vi "SW_Add_or_Modify_Reward_Condition.vi"(6 "IO parameters cluster":T1, 7 "Add or Modify?":enum16{"Add", "Modify"}(ring), 8 "error in (no error)":T15, 9 "Main Tree Control in":refnum<vi>, 10 "Calibration parameters":T13={"Timing calibration sw/hw"=1.0, "True FPS"=80.0, "True frame time, s"=0.0125, "Disp. calibration info"=[]} {"True frame time, s" format="%.10g"; "Disp. calibration info"."Speed, µl per ms" format="%.3g"; "True FPS" format="%.10g"; "Timing calibration sw/hw" format="%.10g"}, 11 "Array of conditions in":T12 {"Specifier(s)"."Validity criteria(s)"."Validity value" min=0.0 step=0.1 format="%.2g"; "Specifier(s)"."Value" step=1.0 format="%#.2g"}) -> (0 "error out":T15, 1 "Main Tree Control out":refnum<vi>, 3 "Array of conditions out":T12 {"Specifier(s)"."Validity criteria(s)"."Validity value" min=0.0 step=0.1 format="%.2g"; "Specifier(s)"."Value" step=1.0 format="%#.2g"})   [LabVIEW 2018, in "Tracker.lvlib"]
uses:
  Tracker.lvlib
  Controls/CTL_Conditions_Array.ctl
  Controls/CTL_Conditions_Cluster.ctl
  Controls/CTL_Condition_type.ctl
  Controls/CTL_Comparison_type.ctl
  Controls/CTL_Validity_check_criteria.ctl
  Controls/CTL_Response_info.ctl
  Controls/CTL_Condition_response_type.ctl
  Controls/CTL_Reponse_port_info.ctl
  Controls/CTL_Calibration_parameters.ctl
  Controls/CTL_Dispenser_calibration_info.ctl
  Controls/CTL_IO_params_cluster.ctl
  <vilib>/Utility/miscctls.llb/LVPointTypeDef.ctl
  Controls/CTL_Conditions_build_parameters_in.ctl
panel:
  out "Local tree ref":refnum<vi>
  in  "Discard and exit":bool
  in  "Reset Button":bool
  out "Index of selected condition":i32
  out "Has been set":bool
  in  "Specifiers On/Off":T2
  in  "Save and exit":bool
  out "Validity criteria(s)":T4(array[cluster])
  out "Subcondition":T5={"Enabled"=FALSE, "Name"="", "Specifier(s)"=[], "Response"={"Response type"=enum."Air puff", "TTL port"=enum."Port 1", "TTL pulse length, ms"=0.0}, "Has been set"=FALSE} caption="Condition" {"Specifier(s)"."Validity criteria(s)"."Validity value" min=0.0 step=0.1 format="%.2g"; "Specifier(s)"."Value" step=1.0 format="%#.2g"}
  in  "TTL pulse length":dbl caption="Puff length, ms"
  in  "TTL port":T10
  in  "Response type":T9=enum."Air puff"
  in  "Valid for, units":dbl caption="Has been True for, units" format="%.2g"
  in  "Validity Enabled":bool caption="Enabled"
  in  "SC. Validity Criteria":T3 caption="Validity Criteria"
  in  "Compare against":dbl
  in  "Comparison type":T7
  in  "SubCondition type":T6
  in  "Subcondition #":i32(slide)=5 min=1 max=5 step=1 scale=5.0..1.0
  in  "Specifier(s)":T11(array[cluster])
  in  "C. Name":string caption="Condition Name"
  out "Cond. work index":i32
  in  "C. Enabled":bool caption="Enabled"
  out "Review changes before save":string(tree) caption="Reward and stimulation out"
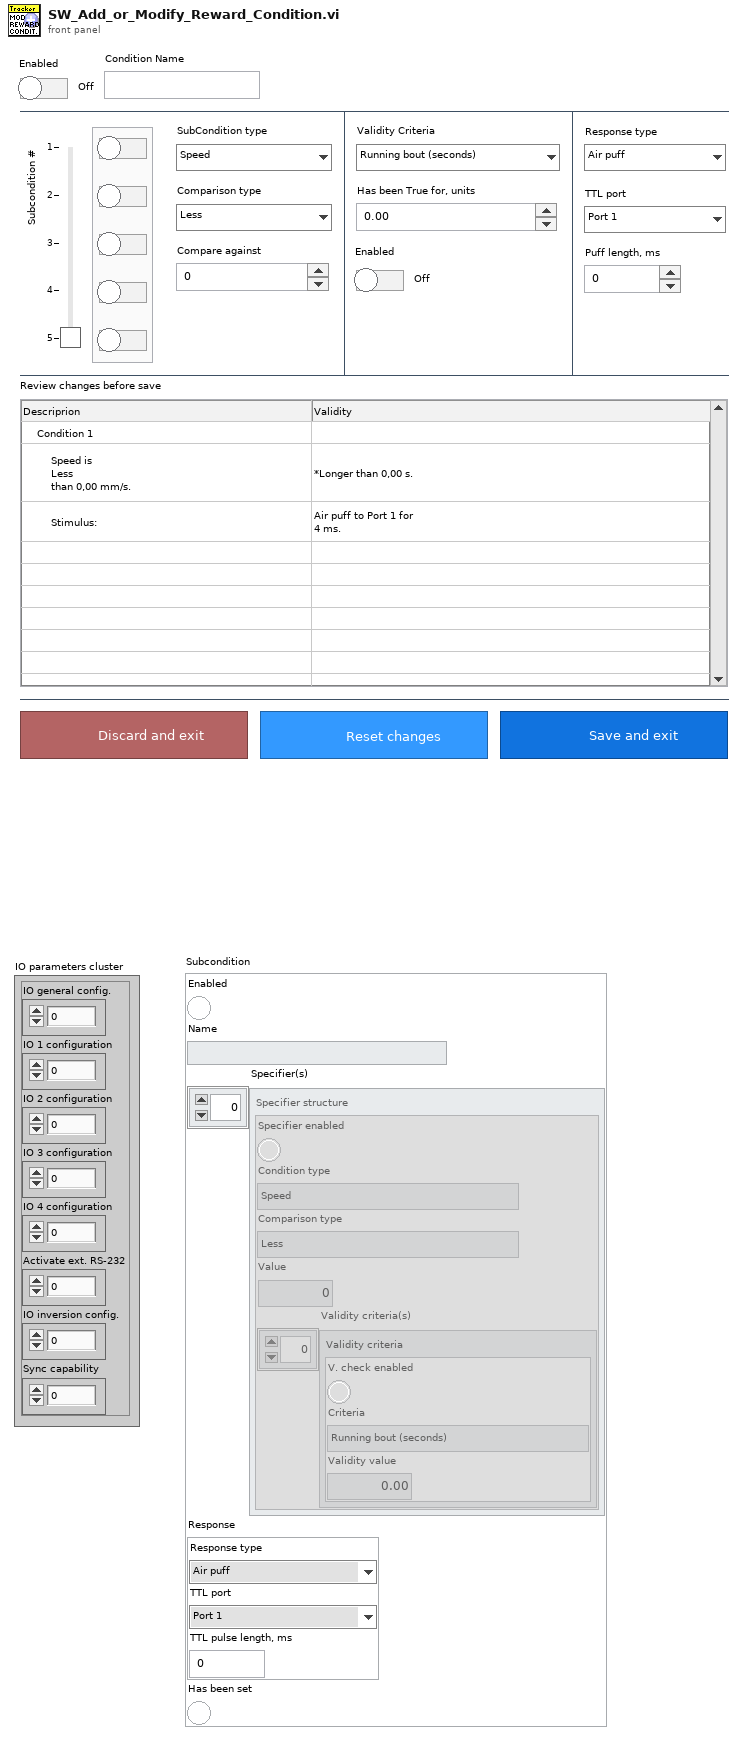
[diagram p1: front panel]
types:
  T1 = typedef "Tracker.lvlib/CTL_IO_params_cluster.ctl" = cluster{"IO general config.":u16, "IO 1 configuration":u16, "IO 2 configuration":u16, "IO 3 configuration":u16, "IO 4 configuration":u16, "Activate ext. RS-232":u16, "IO inversion config.":u16, "Sync capability":u8}
  T2 = cluster{"Specifier on/off":bool, "Specifier on/off 2":bool, "Specifier on/off 3":bool, "Specifier on/off 4":bool, "Specifier on/off 5":bool}
  T3 = typedef "Tracker.lvlib/CTL_Validity_check_criteria.ctl" = enum16{"Running bout (seconds)", "Running bout (meters)"}
  T4 = cluster{"V. check enabled":bool, "Criteria":T3, "Validity value":dbl}[]
  T5 = typedef "Tracker.lvlib/CTL_Conditions_Cluster.ctl" = cluster{"Enabled":bool, "Name":string, "Specifier(s)":cluster{"Specifier enabled":bool, "Condition type":T6, "Comparison type":T7, "Value":dbl, "Validity criteria(s)":cluster{"V. check enabled":bool, "Criteria":T3, "Validity value":dbl}[]}[], "Response":T8, "Has been set":bool}
  T6 = typedef "Tracker.lvlib/CTL_Condition_type.ctl" = enum16{"Speed", "Zone", "Angle to wall"}
  T7 = typedef "Tracker.lvlib/CTL_Comparison_type.ctl" = enum16{"Less", "Less or Equal", "Equal", "Greater or Equal", "Greater", "Not Equal"}
  T8 = typedef "CTL_Response_info.ctl" = cluster{"Response type":T9, "TTL port":T10, "TTL pulse length, ms":dbl}
  T9 = typedef "Tracker.lvlib/CTL_Condition_response_type.ctl" = enum16{"None", "Air puff", "Liquid reward"}
  T10 = typedef "CTL_Reponse_port_info.ctl" = enum16{"Port 1", "Port 2", "Port 3", "Port 4"}
  T11 = cluster{"Specifier enabled":bool, "Condition type":T6, "Comparison type":T7, "Value":dbl, "Validity criteria(s)":cluster{"V. check enabled":bool, "Criteria":T3, "Validity value":dbl}[]}[]
  T12 = typedef "Tracker.lvlib/CTL_Conditions_Array.ctl" = T5[]
  T13 = typedef "Tracker.lvlib/CTL_Calibration_parameters.ctl" = cluster{"Timing calibration sw/hw":dbl, "True FPS":dbl, "True frame time, s":dbl, "Disp. calibration info":T14}
  T14 = typedef "Tracker.lvlib/CTL_Dispenser_calibration_info.ctl" = cluster{"Channel":u8, "Speed, µl per ms":dbl}[]
  T15 = cluster{"Boolean Round":bool, "code":i32, "source":string}
  T16 = typedef "LVPointTypeDef.ctl" = cluster{"Horizontal":i16, "Vertical":i16}
  T17 = typedef "Tracker.lvlib/CTL_Conditions_build_parameters_in.ctl" = cluster{"TreeControl in":refnum<vi>, "TTL pulse length ref in":refnum<vi>, "Array of conditions in":T12, "Condition working index":i32, "Subcondition #":i32, "Calibration parameters":T13}
  T18 = typedef "Tracker.lvlib/CTL_Conditions_build_parameters_out.ctl" = cluster{"TreeControl ref out":refnum<vi>, "SubCondition":T5, "C. Enabled":bool, "C. Name":string, "Specifier(s)":cluster{"Specifier enabled":bool, "Condition type":T6, "Comparison type":T7, "Value":dbl, "Validity criteria(s)":cluster{"V. check enabled":bool, "Criteria":T3, "Validity value":dbl}[]}[], "Has been set":bool, "Condition type":T6, "Comparison type":T7, "Compare against value":dbl, "Validity criteria(s)":cluster{"V. check enabled":bool, "Criteria":T3, "Validity value":dbl}[], "V. check enabled":bool, "Validity criteria":T3, "Validity value":dbl, "Specifiers On/Off":cluster{"[0]":bool, "[1]":bool, "[2]":bool, "[3]":bool, "[4]":bool}, "Response type":T9, "TTL port":T10, "TTL pulse length, ms out":dbl}
  T19 = cluster{"[0]":bool, "[1]":bool, "[2]":bool, "[3]":bool, "[4]":bool}
  T20 = cluster{"Specifier enabled":bool, "Condition type":T6, "Comparison type":T7, "Value":dbl, "Validity criteria(s)":cluster{"V. check enabled":bool, "Criteria":T3, "Validity value":dbl}[]}
  T21 = cluster{"V. check enabled":bool, "Criteria":T3, "Validity value":dbl}
  T22 = cluster{"Specifiers On/Off[0]":bool, "Specifiers On/Off[1]":bool, "Specifiers On/Off[2]":bool, "Specifiers On/Off[3]":bool, "Specifiers On/Off[4]":bool}
  T23 = cluster{"Validity Enabled":bool, "SC. Validity Criteria":T3, "Valid for, units":dbl}
  T24 = cluster{"Response type":T9, "TTL port":T10, "TTL pulse length, ms out":dbl}
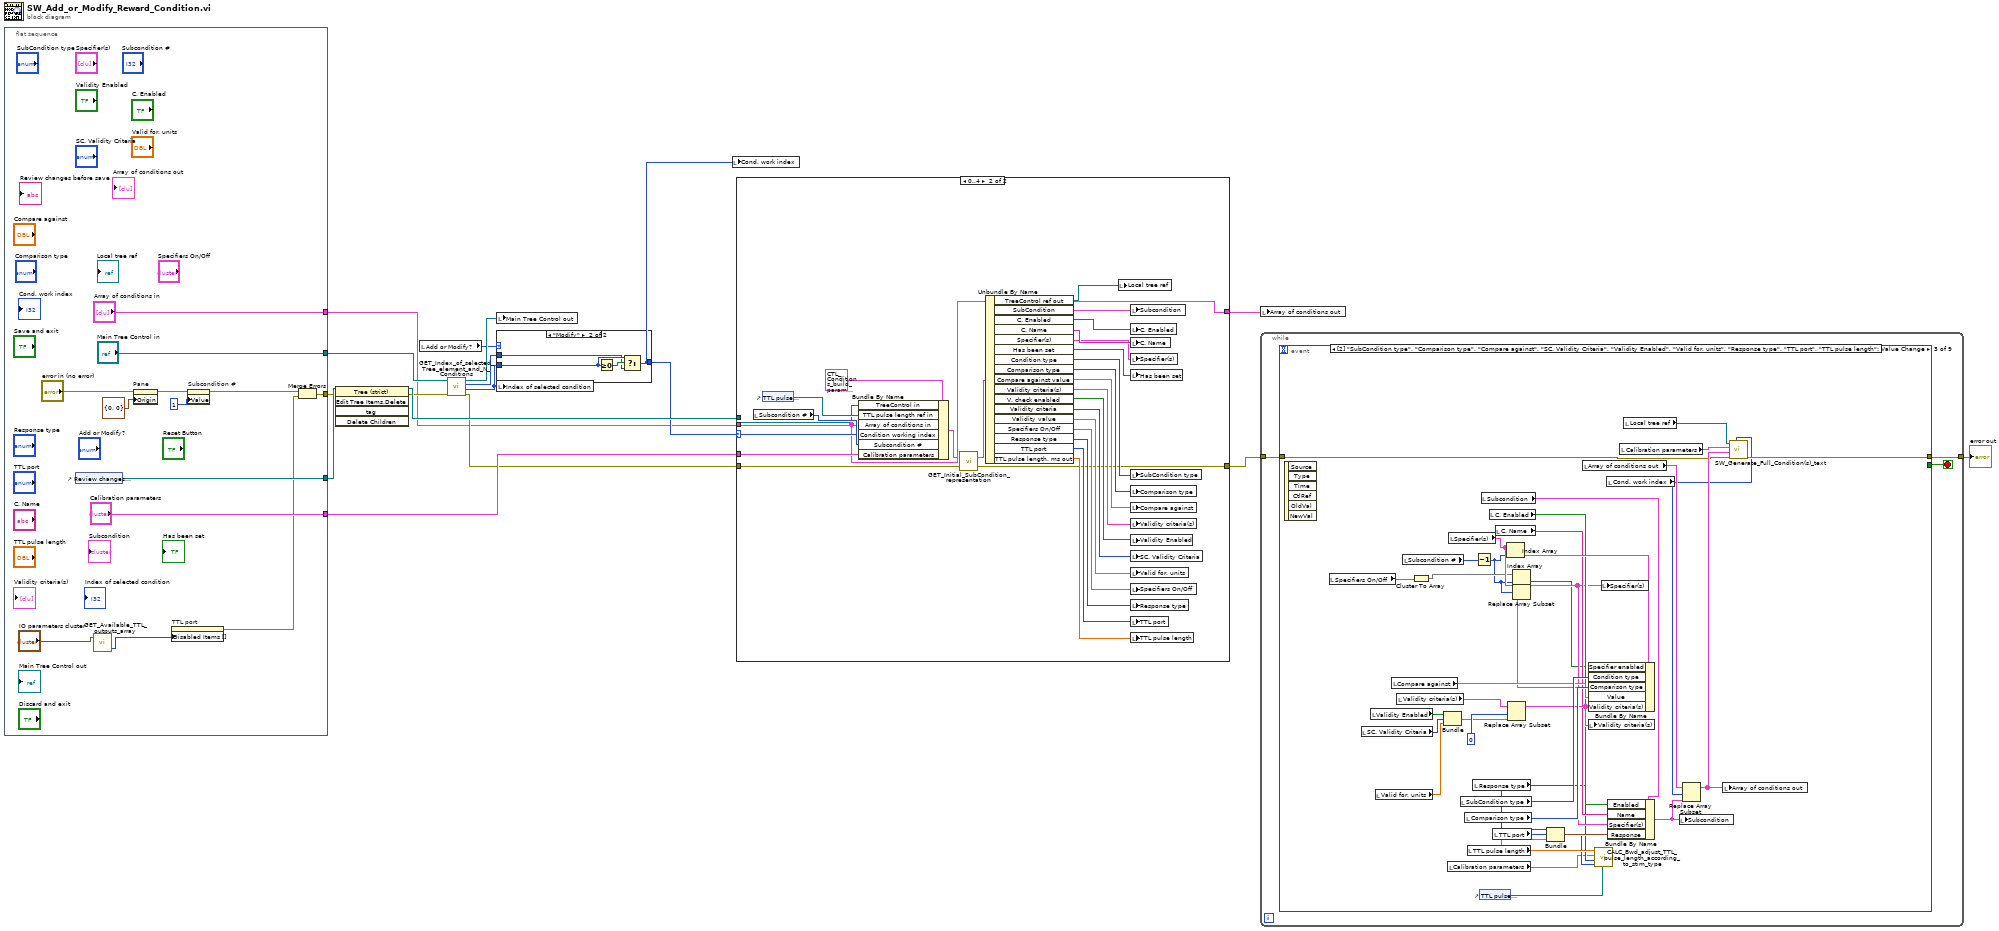
[diagram p0: block diagram]
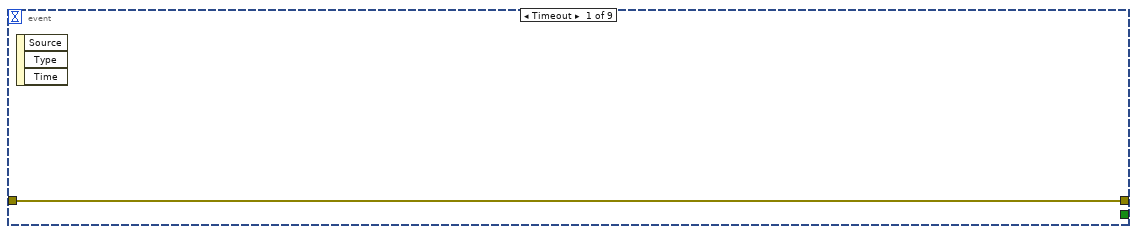
[diagram p4: hidden frame]
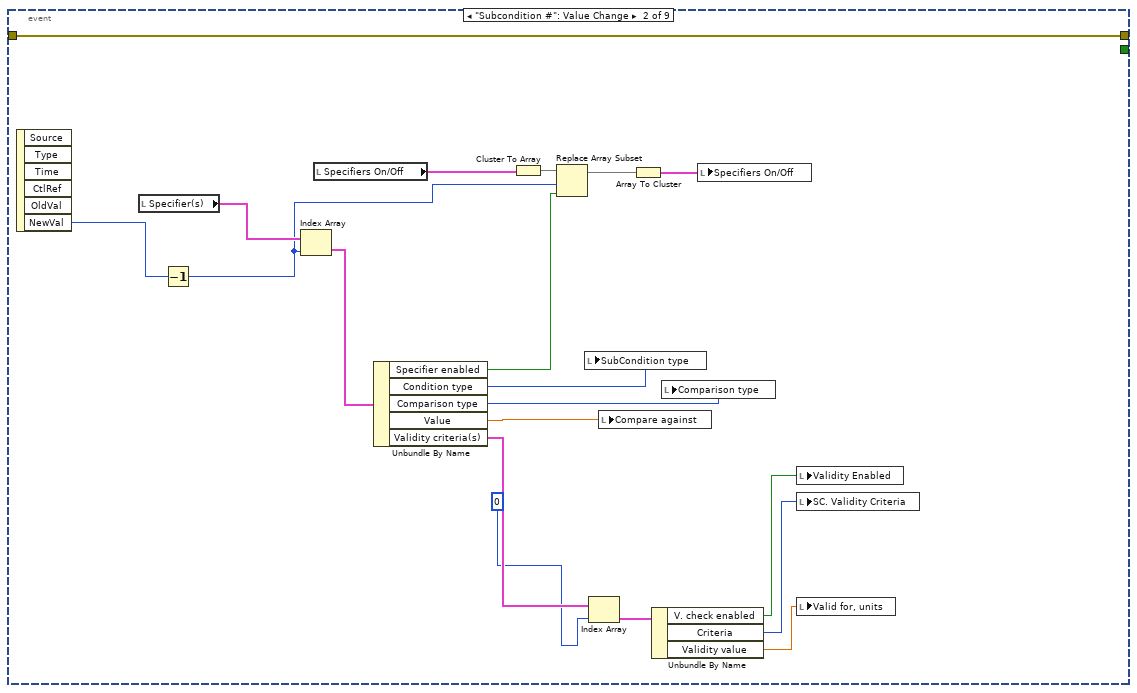
[diagram p5: hidden frame]
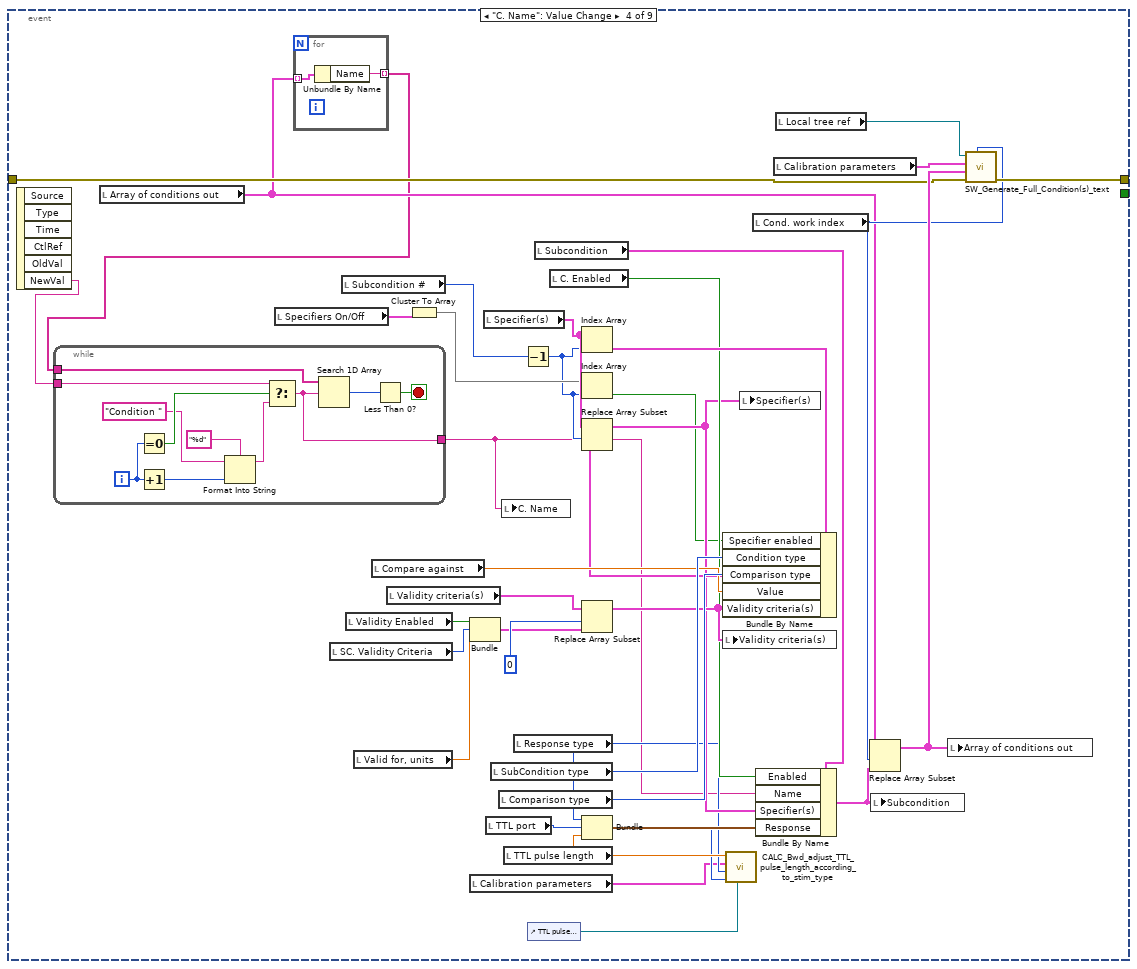
[diagram p6: hidden frame]
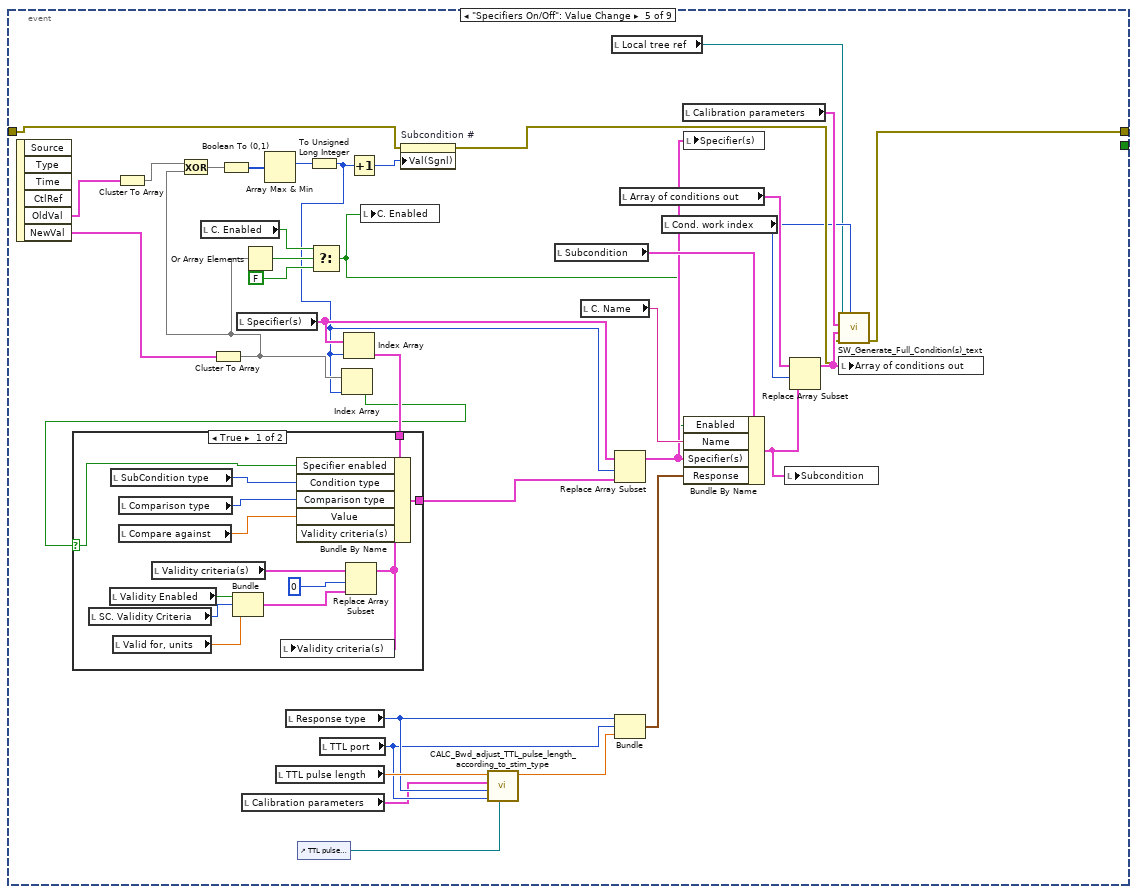
[diagram p7: hidden frame]
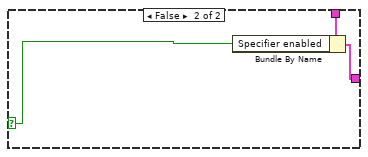
[diagram p8: hidden frame]
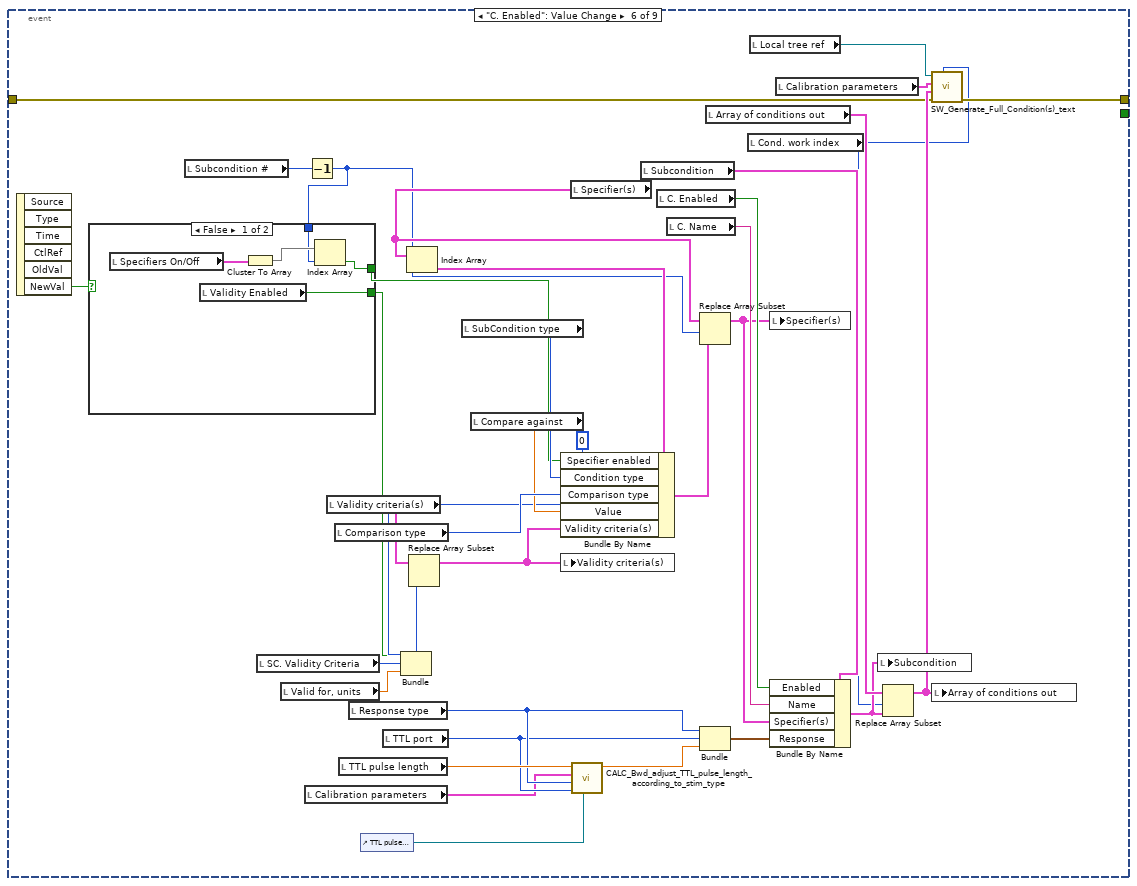
[diagram p9: hidden frame]
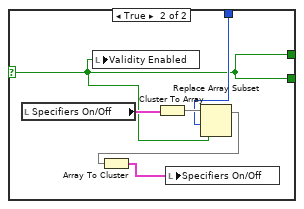
[diagram p10: hidden frame]
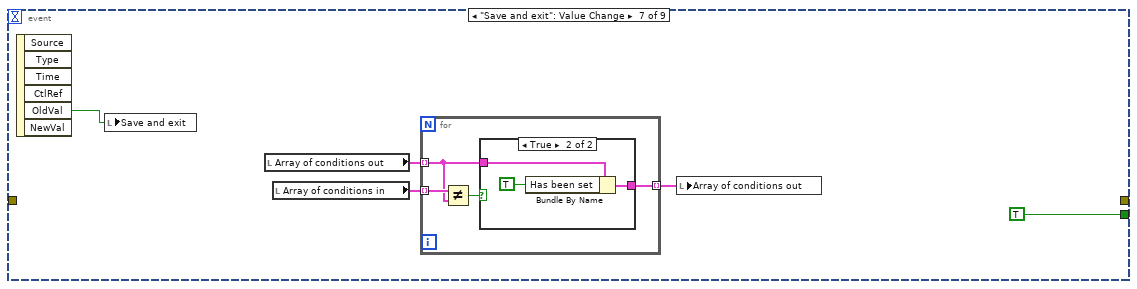
[diagram p11: hidden frame]
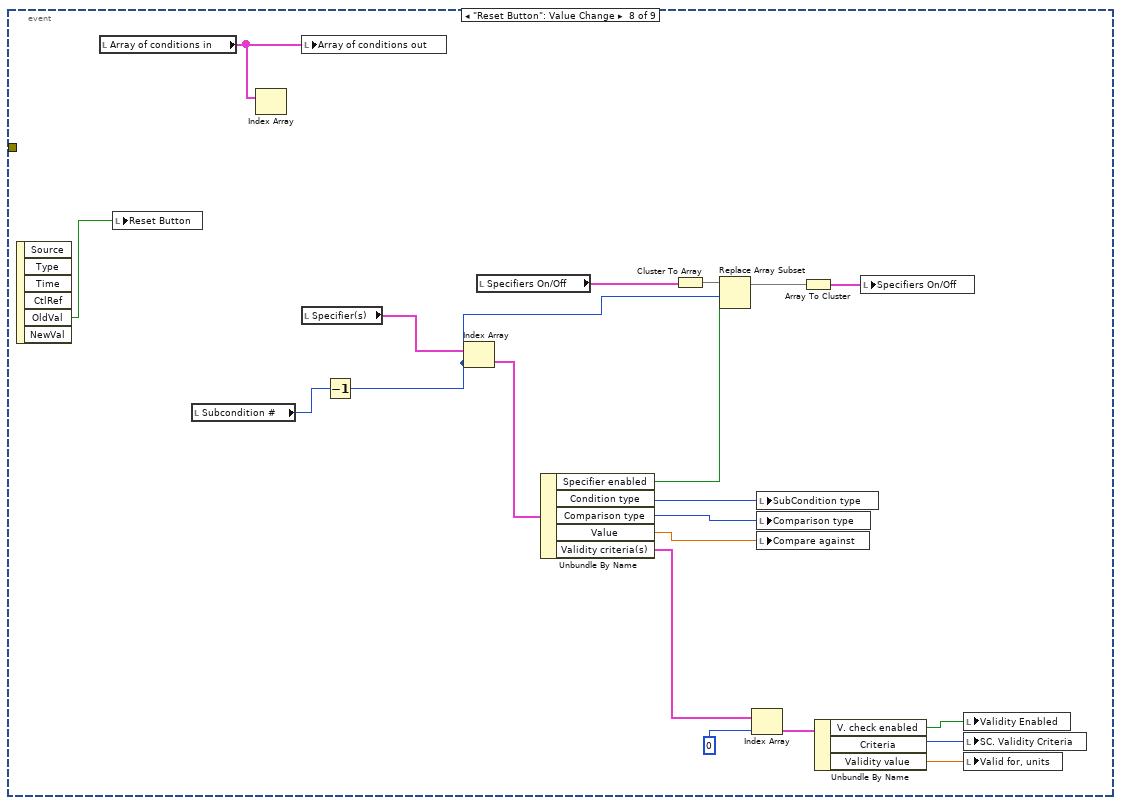
[diagram p13: hidden frame]
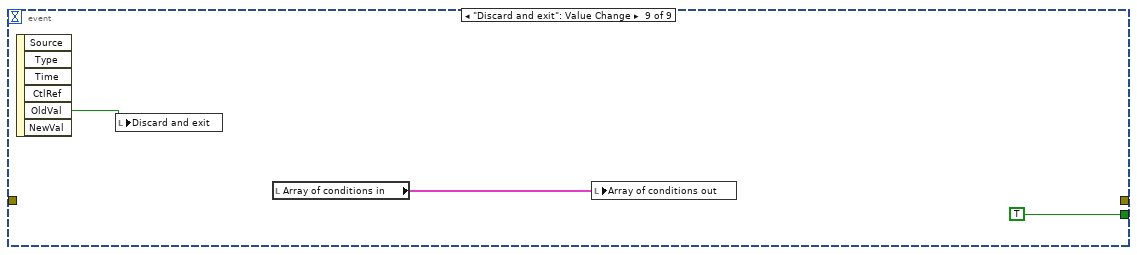
[diagram p14: hidden frame]
diagram:
  n1 = flat-sequence {
    tunnel: [w19] -> w14
    tunnel: [w27] -> w15
    tunnel: ["Main Tree Control in"] -> w4
    tunnel: ["Array of conditions in"] -> w1
    tunnel: ["Calibration parameters"] -> w12
    frame #0 {
      n2 = control-ref of="Review changes before save"() -> (w27:refnum<vi>)
      n3 = call "GET_Available_TTL_outputs_array.vi"("IO parameters cluster"="IO parameters cluster") -> ("Disabled items"=w17:i32[])  [unwired: 2 in, 1 out]
      n4 = property on="Pane" class="Pane"(error in="error in (no error)", "Origin"=T16 {"Horizontal"=0, "Vertical"=0}) -> (error out=w23:errorcluster)  [unwired: 1 in, 1 out]
      n5 = property on="TTL port" class="Enum (strict)"("Disabled Items []"=w17) -> (error out=w18:errorcluster)  [unwired: 2 in, 1 out]
      n6 = property on="Subcondition #" class="Slide (strict)"(error in=w23, "Value"=1 ("Subcondition #")) -> (error out=w22:errorcluster)  [unwired: 1 in, 1 out]
      n7 = Merge Errors(w22, w18) -> (w19:errorcluster)
    }
  }
  n8 = invoke class="Tree (strict)" method="Edit Tree Items.Delete"(reference=w15, error in=w14) -> (reference out=w11:refnum<vi>, error out=w5:errorcluster)  [unwired: 3 in, 3 out]
  n9 = local read "Add or Modify?"() -> (w7:enum16{"Add", "Modify"})
  n10 = call "GET_Index_of_selected_Tree_element_and_N_Conditions.vi"("error in (no error)"=w5, "TreeControl in"=w4) -> ("error out"=w8:errorcluster, "Index of selected element"=w2:i32, "Amount of conditions"=w3:i32, "TreeControl out"=w9:refnum<vi>)  [unwired: 6 in]
  n11 = local write "Main Tree Control out"(w9) -> ()
  n12 = case shown="\"Modify\"" w7 {
    tunnel: w3 -> [w30 w31]
    tunnel: w2 -> [_ w32]
    tunnel: [w30 w34] -> w6
    frame "Add", Default {
    }
    frame "Modify" {
      n13 = Greater Or Equal To 0?(x=w32) -> (x >= 0?=w33:bool)
      n14 = Select(t=w32, s=w33, f=w31) -> (s? t:f=w34:i32)
    }
  }
  n15 = local write "Index of selected condition"(w2) -> ()
  n16 = local write "Cond. work index"(w6) -> ()
  n17 = case shown="0..4" w6 {
    selector: w6 -> [_ w60]
    tunnel: w1 -> [w36 w58]
    tunnel: [w36 w58] -> w13
    tunnel: w8 -> [w35 w64]
    tunnel: w12 -> [_ w61]
    tunnel: w11 -> [_ w59]
    tunnel: [w35 w39] -> w10
    frame 5.., Default {
    }
    frame 0..4 {
      n18 = local read "Subcondition #"() -> (w62:i32)
      n19 = control-ref of="TTL pulse length"() -> (w63:refnum<vi>)
      n20 = Bundle By Name(cluster=T17 {"TreeControl in"=refnum, "TTL pulse length ref in"=refnum, "Array of conditions in"=[], "Condition working index"=0, "Subcondition #"=0, "Calibration parameters"={"Timing calibration sw/hw"=0.0, "True FPS"=0.0, "True frame time, s"=0.0, "Disp. calibration info"=[]}} ("Input parameters cluster"), "TreeControl in"=w59, "TTL pulse length ref in"=w63, "Array of conditions in"=w58, "Condition working index"=w60, "Subcondition #"=w62, "Calibration parameters"=w61) -> (w57:T17)
      n21 = call "GET_Initial_SubCondition_representation.vi"("error in (no error)"=w64, "Input parameters cluster"=w57) -> ("error out"=w39:errorcluster, "Output parameters cluster"=w56:T18)
      n22 = Unbundle By Name(w56) -> ("TreeControl ref out"=w38:refnum<vi>, "SubCondition"=w51:T5, "C. Enabled"=w50:bool, "C. Name"=w49:string, "Specifier(s)"=w48:T11, "Has been set"=w40:bool, "Condition type"=w47:T6, "Comparison type"=w41:T7, "Compare against value"=w43:dbl, "Validity criteria(s)"=w42:T4, "V. check enabled"=w45:bool, "Validity criteria"=w46:T3, "Validity value"=w44:dbl, "Specifiers On/Off"=w52:T19, "Response type"=w55:T9, "TTL port"=w53:T10, "TTL pulse length, ms out"=w54:dbl)
      n23 = local write "Local tree ref"(w38) -> ()
      n24 = local write "Subcondition"(w51) -> ()
      n25 = local write "C. Enabled"(w50) -> ()
      n26 = local write "C. Name"(w49) -> ()
      n27 = local write "Specifier(s)"(w48) -> ()
      n28 = local write "Has been set"(w40) -> ()
      n29 = local write "SubCondition type"(w47) -> ()
      n30 = local write "Comparison type"(w41) -> ()
      n31 = local write "Compare against"(w43) -> ()
      n32 = local write "Validity criteria(s)"(w42) -> ()
      n33 = local write "Validity Enabled"(w45) -> ()
      n34 = local write "SC. Validity Criteria"(w46) -> ()
      n35 = local write "Valid for, units"(w44) -> ()
      n36 = local write "Specifiers On/Off"(w52) -> ()
      n37 = local write "Response type"(w55) -> ()
      n38 = local write "TTL port"(w53) -> ()
      n39 = local write "TTL pulse length"(w54) -> ()
    }
  }
  n40 = local write "Array of conditions out"(w13) -> ()
  n41 = while {
    tunnel: w10 -> [w67]
    tunnel: [w66] -> w16
    stop <- w65 stop-if-true
    n42 = event shown="[2] \"SubCondition type\", \"Comparison type\", \"Compare against\", \"SC. Validity Criteria\", \"Validity Enabled\", \"Valid for, units\", \"Response type\", \"TTL port\", \"TTL pulse length\": Value Change" {
      selector: _ -> [_ _ _ _ _ _ _ _ _]
      dyn-events: _ -> [_ _ _ _ _ _ _ _ _]
      timeout: _ -> [_ _ _ _ _ _ _ _ _]
      tunnel: w67 -> [w68 w86 w102 w143 w183 w243 _ _ _]
      tunnel: [w68 w86 w101 w142 w201 w242 _ _ _] -> w66
      tunnel: [_ _ _ _ _ _ TRUE _ TRUE] -> w65
      event Timeout {
        n43 = event-data() -> ()  [unwired: 1 in, 3 out]
      }
      event "Subcondition #": Value Change {
        n44 = event-data() -> ("NewVal"=w87:i32)  [unwired: 1 in, 5 out]
        n45 = local read "Specifier(s)"() -> (w85:T11)
        n46 = Decrement(x=w87) -> (x-1=w69:i32)
        n47 = Index Array(array=w85, index=w69) -> (element=w84:T20)
        n48 = local read "Specifiers On/Off"() -> (w74:T2)
        n49 = Unbundle By Name(w84) -> ("Specifier enabled"=w70:bool, "Condition type"=w83:T6, "Comparison type"=w82:T7, "Value"=w81:dbl, "Validity criteria(s)"=w80:T4)
        n50 = Cluster To Array(cluster=w74) -> (array=w73:bool[])
        n51 = Replace Array Subset(array=w73, new element=w70, index=w69) -> (w72:bool[])
        n52 = local write "SubCondition type"(w83) -> ()
        n53 = Index Array(array=w80, index=0) -> (element=w78:T21)
        n54 = local write "Compare against"(w81) -> ()
        n55 = Array To Cluster(array=w72) -> (cluster=w71:T22)
        n56 = Unbundle By Name(w78) -> ("V. check enabled"=w76:bool, "Criteria"=w77:T3, "Validity value"=w75:dbl)
        n57 = local write "Comparison type"(w82) -> ()
        n58 = local write "Specifiers On/Off"(w71) -> ()
        n59 = local write "Validity Enabled"(w76) -> ()
        n60 = local write "SC. Validity Criteria"(w77) -> ()
        n61 = local write "Valid for, units"(w75) -> ()
      }
      event "Compare against", "Validity Enabled", "Valid for, units", "TTL pulse length": Value Change {
        n62 = event-data() -> ()  [unwired: 1 in, 6 out]
        n63 = local read "Specifiers On/Off"() -> (w94:T2)
        n64 = local read "SC. Validity Criteria"() -> (w117:T3)
        n65 = local read "Validity Enabled"() -> (w118:bool)
        n66 = local read "Valid for, units"() -> (w116:dbl)
        n67 = local read "Compare against"() -> (w121:dbl)
        n68 = local read "Validity criteria(s)"() -> (w120:T4)
        n69 = local read "Subcondition #"() -> (w89:i32)
        n70 = Cluster To Array(cluster=w94) -> (array=w93:bool[])
        n71 = Bundle("Validity Enabled"=w118, "SC. Validity Criteria"=w117, "Valid for, units"=w116) -> (w115:T23)  [unwired: 1 in]
        n72 = local read "Calibration parameters"() -> (w96:T13)
        n73 = local read "Specifier(s)"() -> (w113:T11)
        n74 = local read "SubCondition type"() -> (w123:T6)
        n75 = local read "Comparison type"() -> (w122:T7)
        n76 = local read "TTL pulse length"() -> (w100:dbl)
        n77 = local read "Response type"() -> (w99:T9)
        n78 = Decrement(x=w89) -> (x-1=w91:i32)
        n79 = control-ref of="TTL pulse length"() -> (w95:refnum<vi>)
        n80 = local read "Subcondition"() -> (w108:T5)
        n81 = local read "C. Enabled"() -> (w109:bool)
        n82 = local read "TTL port"() -> (w98:T10)
        n83 = local read "C. Name"() -> (w110:string)
        n84 = Index Array(array=w113, index=w91) -> (element=w124:T20)
        n85 = Replace Array Subset(array=w120, new element=w115, index=0) -> (w114:T4)
        n86 = Index Array(array=w93, index=w91) -> (element=w92:bool)
        n87 = local read "Array of conditions out"() -> (w106:T12)
        n88 = Bundle By Name(cluster=w124, "Specifier enabled"=w92, "Condition type"=w123, "Comparison type"=w122, "Value"=w121, "Validity criteria(s)"=w114) -> (w112:T20)
        n89 = Replace Array Subset(array=w113, new element=w112, index=w91) -> (w107:T11)
        n90 = local write "Validity criteria(s)"(w114) -> ()
        n91 = call "CALC_Bwd_adjust_TTL_pulse_length_according_to_stim_type.vi"("TTL pulse length ref in"=w95, "TTL port"=w98, "Response type"=w99, "Calibration parameters"=w96, "TTL pulse length, units, in"=w100) -> ("TTL pulse length, ms out"=w97:dbl)  [unwired: 6 in]
        n92 = Bundle("Response type"=w99, "TTL port"=w98, "TTL pulse length, ms out"=w97) -> (w111:T24)  [unwired: 1 in]
        n93 = local write "Specifier(s)"(w107) -> ()
        n94 = local read "Cond. work index"() -> (w90:i32)
        n95 = Bundle By Name(cluster=w108, "Enabled"=w109, "Name"=w110, "Specifier(s)"=w107, "Response"=w111) -> (w105:T5)
        n96 = local read "Calibration parameters"() -> (w103:T13)
        n97 = local read "Local tree ref"() -> (w88:refnum<vi>)
        n98 = local write "Subcondition"(w105) -> ()
        n99 = Replace Array Subset(array=w106, new element=w105, index=w90) -> (w104:T12)
        n100 = local write "Array of conditions out"(w104) -> ()
        n101 = call "SW_Generate_Full_Condition(s)_text.vi"("Array index to show"=w90, "error in (no error)"=w102, "Array of conditions in"=w104, "Calibration parameters"=w103, "TreeControl ref in"=w88) -> ("error out"=w101:errorcluster)  [unwired: 5 in, 1 out]
      }
      event "C. Name": Value Change {
        n102 = event-data() -> ("NewVal"=w129:string)  [unwired: 1 in, 5 out]
        n103 = local read "Array of conditions out"() -> (w128:T12)
        n104 = local read "Specifiers On/Off"() -> (w135:T2)
        n105 = for {
          tunnel: w128 -> [w165] mode=indexing
          tunnel: [w164] -> w127 mode=indexing
          n106 = Unbundle By Name(w165) -> ("Name"=w164:string)
        }
        n107 = while {
          tunnel: w127 -> [w175]
          tunnel: [w166] -> w126
          tunnel: w129 -> [w167]
          i -> [w169]
          stop <- w174 stop-if-true
          n108 = Equal To 0?(x=w169) -> (x = 0?=w173:bool)
          n109 = Increment(x=w169) -> (x+1=w172:i32)
          n110 = Format Into String(format string="%d", initial string="Condition ", w172) -> (resulting string=w168:string)  [unwired: 1 in, 1 out]
          n111 = Select(t=w167, s=w173, f=w168) -> (s? t:f=w166:string)
          n112 = Search 1D Array(1D array=w175, element=w166) -> (index of element=w176:i32)  [unwired: 1 in]
          n113 = Less Than 0?(x=w176) -> (x < 0?=w174:bool)
        }
        n114 = local read "SC. Validity Criteria"() -> (w156:T3)
        n115 = local read "Subcondition #"() -> (w130:i32)
        n116 = local read "Validity Enabled"() -> (w157:bool)
        n117 = local read "Valid for, units"() -> (w155:dbl)
        n118 = local read "Compare against"() -> (w160:dbl)
        n119 = local read "Validity criteria(s)"() -> (w159:T4)
        n120 = Cluster To Array(cluster=w135) -> (array=w134:bool[])
        n121 = Bundle("Validity Enabled"=w157, "SC. Validity Criteria"=w156, "Valid for, units"=w155) -> (w154:T23)  [unwired: 1 in]
        n122 = local read "Calibration parameters"() -> (w137:T13)
        n123 = local read "Specifier(s)"() -> (w152:T11)
        n124 = local read "TTL port"() -> (w139:T10)
        n125 = local read "SubCondition type"() -> (w162:T6)
        n126 = local read "Comparison type"() -> (w161:T7)
        n127 = local write "C. Name"(w126) -> ()
        n128 = local read "TTL pulse length"() -> (w141:dbl)
        n129 = local read "Response type"() -> (w140:T9)
        n130 = Decrement(x=w130) -> (x-1=w132:i32)
        n131 = control-ref of="TTL pulse length"() -> (w136:refnum<vi>)
        n132 = local read "Subcondition"() -> (w148:T5)
        n133 = local read "C. Enabled"() -> (w149:bool)
        n134 = Index Array(array=w152, index=w132) -> (element=w163:T20)
        n135 = Index Array(array=w134, index=w132) -> (element=w133:bool)
        n136 = Replace Array Subset(array=w159, new element=w154, index=0) -> (w153:T4)
        n137 = Bundle By Name(cluster=w163, "Specifier enabled"=w133, "Condition type"=w162, "Comparison type"=w161, "Value"=w160, "Validity criteria(s)"=w153) -> (w151:T20)
        n138 = Replace Array Subset(array=w152, new element=w151, index=w132) -> (w147:T11)
        n139 = local write "Validity criteria(s)"(w153) -> ()
        n140 = call "CALC_Bwd_adjust_TTL_pulse_length_according_to_stim_type.vi"("TTL pulse length ref in"=w136, "TTL port"=w139, "Response type"=w140, "Calibration parameters"=w137, "TTL pulse length, units, in"=w141) -> ("TTL pulse length, ms out"=w138:dbl)  [unwired: 6 in]
        n141 = Bundle("Response type"=w140, "TTL port"=w139, "TTL pulse length, ms out"=w138) -> (w150:T24)  [unwired: 1 in]
        n142 = local write "Specifier(s)"(w147) -> ()
        n143 = local read "Cond. work index"() -> (w131:i32)
        n144 = Bundle By Name(cluster=w148, "Enabled"=w149, "Name"=w126, "Specifier(s)"=w147, "Response"=w150) -> (w146:T5)
        n145 = local read "Calibration parameters"() -> (w144:T13)
        n146 = local read "Local tree ref"() -> (w125:refnum<vi>)
        n147 = Replace Array Subset(array=w128, new element=w146, index=w131) -> (w145:T12)
        n148 = local write "Subcondition"(w146) -> ()
        n149 = local write "Array of conditions out"(w145) -> ()
        n150 = call "SW_Generate_Full_Condition(s)_text.vi"("Array index to show"=w131, "error in (no error)"=w143, "Array of conditions in"=w145, "Calibration parameters"=w144, "TreeControl ref in"=w125) -> ("error out"=w142:errorcluster)  [unwired: 5 in, 1 out]
      }
      event "Specifiers On/Off": Value Change {
        n151 = event-data() -> ("OldVal"=w189:T2, "NewVal"=w190:T2)  [unwired: 1 in, 4 out]
        n152 = Cluster To Array(cluster=w189) -> (array=w188:bool[])
        n153 = local read "C. Enabled"() -> (w192:bool)
        n154 = Cluster To Array(cluster=w190) -> (array=w187:bool[])
        n155 = Exclusive Or(1:w187, 2:w188) -> (0:w186:bool[])
        n156 = Boolean To (0,1)(Boolean=w186) -> (0, 1=w185:i16[])
        n157 = local read "Specifier(s)"() -> (w211:T11)
        n158 = local read "Calibration parameters"() -> (w196:T13)
        n159 = Or Array Elements(Boolean array=w187) -> (logical OR=w194:bool)
        n160 = Array Max & Min(array=w185) -> (max index (indices)=w184:i32)  [unwired: 3 out]
        n161 = local read "TTL pulse length"() -> (w200:dbl)
        n162 = local read "Response type"() -> (w199:T9)
        n163 = control-ref of="TTL pulse length"() -> (w195:refnum<vi>)
        n164 = To Unsigned Long Integer(number=w184) -> (unsigned 32bit integer=w180:u32)
        n165 = Select(t=w192, s=w194, f=FALSE) -> (s? t:f=w191:bool)
        n166 = local read "TTL port"() -> (w198:T10)
        n167 = Index Array(array=w187, index=w180) -> (element=w181:bool)
        n168 = Index Array(array=w211, index=w180) -> (element=w212:T20)
        n169 = case shown="True" w181 {
          selector: w181 -> [w213 w226]
          tunnel: w212 -> [w225 w228]
          tunnel: [w214 w227] -> w210
          frame True {
            n170 = local read "SC. Validity Criteria"() -> (w218:T3)
            n171 = local read "Validity Enabled"() -> (w219:bool)
            n172 = local read "SubCondition type"() -> (w224:T6)
            n173 = local read "Valid for, units"() -> (w217:dbl)
            n174 = local read "Comparison type"() -> (w223:T7)
            n175 = local read "Compare against"() -> (w222:dbl)
            n176 = local read "Validity criteria(s)"() -> (w221:T4)
            n177 = Bundle("Validity Enabled"=w219, "SC. Validity Criteria"=w218, "Valid for, units"=w217) -> (w216:T23)  [unwired: 1 in]
            n178 = Replace Array Subset(array=w221, new element=w216, index=0) -> (w215:T4)
            n179 = local write "Validity criteria(s)"(w215) -> ()
            n180 = Bundle By Name(cluster=w225, "Specifier enabled"=w213, "Condition type"=w224, "Comparison type"=w223, "Value"=w222, "Validity criteria(s)"=w215) -> (w214:T20)
          }
          frame False {
            n181 = Bundle By Name(cluster=w228, "Specifier enabled"=w226) -> (w227:T20)
          }
        }
        n182 = Increment(x=w180) -> (x+1=w179:u32)
        n183 = local write "C. Enabled"(w191) -> ()
        n184 = property on="Subcondition #" class="Slide (strict)"(error in=w183, "Val(Sgnl)"=w179) -> (error out=w182:errorcluster)  [unwired: 1 in, 1 out]
        n185 = call "CALC_Bwd_adjust_TTL_pulse_length_according_to_stim_type.vi"("TTL pulse length ref in"=w195, "TTL port"=w198, "Response type"=w199, "Calibration parameters"=w196, "TTL pulse length, units, in"=w200) -> ("TTL pulse length, ms out"=w197:dbl)  [unwired: 6 in]
        n186 = local read "Subcondition"() -> (w207:T5)
        n187 = local read "C. Name"() -> (w208:string)
        n188 = local read "Local tree ref"() -> (w177:refnum<vi>)
        n189 = Replace Array Subset(array=w211, new element=w210, index=w180) -> (w206:T11)
        n190 = Bundle("Response type"=w199, "TTL port"=w198, "TTL pulse length, ms out"=w197) -> (w209:T24)  [unwired: 1 in]
        n191 = local read "Array of conditions out"() -> (w205:T12)
        n192 = local read "Cond. work index"() -> (w178:i32)
        n193 = local read "Calibration parameters"() -> (w202:T13)
        n194 = local write "Specifier(s)"(w206) -> ()
        n195 = Bundle By Name(cluster=w207, "Enabled"=w191, "Name"=w208, "Specifier(s)"=w206, "Response"=w209) -> (w204:T5)
        n196 = local write "Subcondition"(w204) -> ()
        n197 = Replace Array Subset(array=w205, new element=w204, index=w178) -> (w203:T12)
        n198 = call "SW_Generate_Full_Condition(s)_text.vi"("Array index to show"=w178, "error in (no error)"=w182, "Array of conditions in"=w203, "Calibration parameters"=w202, "TreeControl ref in"=w177) -> ("error out"=w201:errorcluster)  [unwired: 5 in, 1 out]
        n199 = local write "Array of conditions out"(w203) -> ()
      }
      event "C. Enabled": Value Change {
        n200 = event-data() -> ("NewVal"=w235:bool)  [unwired: 1 in, 5 out]
        n201 = local read "Subcondition #"() -> (w231:i32)
        n202 = local read "SC. Validity Criteria"() -> (w258:T3)
        n203 = local read "Valid for, units"() -> (w257:dbl)
        n204 = local read "Calibration parameters"() -> (w237:T13)
        n205 = Decrement(x=w231) -> (x-1=w232:i32)
        n206 = case shown="False" w235 {
          selector: w235 -> [_ w272]
          tunnel: [w266 w272] -> w234
          tunnel: [w269 w272] -> w233
          tunnel: w232 -> [w265 w273]
          frame False {
            n207 = local read "Specifiers On/Off"() -> (w268:T2)
            n208 = local read "Validity Enabled"() -> (w269:bool)
            n209 = Cluster To Array(cluster=w268) -> (array=w267:bool[])
            n210 = Index Array(array=w267, index=w265) -> (element=w266:bool)
          }
          frame True {
            n211 = local read "Specifiers On/Off"() -> (w275:T2)
            n212 = local write "Validity Enabled"(w272) -> ()
            n213 = Cluster To Array(cluster=w275) -> (array=w274:bool[])
            n214 = Replace Array Subset(array=w274, new element=w272, index=w273) -> (w271:bool[])
            n215 = Array To Cluster(array=w271) -> (cluster=w270:T22)
            n216 = local write "Specifiers On/Off"(w270) -> ()
          }
        }
        n217 = local read "Validity criteria(s)"() -> (w260:T4)
        n218 = local read "Comparison type"() -> (w262:T7)
        n219 = local read "TTL pulse length"() -> (w241:dbl)
        n220 = local read "Response type"() -> (w240:T9)
        n221 = control-ref of="TTL pulse length"() -> (w236:refnum<vi>)
        n222 = local read "TTL port"() -> (w239:T10)
        n223 = Bundle("Validity Enabled"=w233, "SC. Validity Criteria"=w258, "Valid for, units"=w257) -> (w256:T23)  [unwired: 1 in]
        n224 = Replace Array Subset(array=w260, new element=w256, index=0) -> (w255:T4)
        n225 = local read "SubCondition type"() -> (w263:T6)
        n226 = local read "Compare against"() -> (w261:dbl)
        n227 = local write "Validity criteria(s)"(w255) -> ()
        n228 = local read "Specifier(s)"() -> (w254:T11)
        n229 = Index Array(array=w254, index=w232) -> (element=w264:T20)
        n230 = Bundle By Name(cluster=w264, "Specifier enabled"=w234, "Condition type"=w263, "Comparison type"=w262, "Value"=w261, "Validity criteria(s)"=w255) -> (w253:T20)
        n231 = call "CALC_Bwd_adjust_TTL_pulse_length_according_to_stim_type.vi"("TTL pulse length ref in"=w236, "TTL port"=w239, "Response type"=w240, "Calibration parameters"=w237, "TTL pulse length, units, in"=w241) -> ("TTL pulse length, ms out"=w238:dbl)  [unwired: 6 in]
        n232 = local read "Subcondition"() -> (w249:T5)
        n233 = local read "C. Enabled"() -> (w250:bool)
        n234 = local read "C. Name"() -> (w251:string)
        n235 = Replace Array Subset(array=w254, new element=w253, index=w232) -> (w248:T11)
        n236 = Bundle("Response type"=w240, "TTL port"=w239, "TTL pulse length, ms out"=w238) -> (w252:T24)  [unwired: 1 in]
        n237 = local read "Array of conditions out"() -> (w247:T12)
        n238 = local read "Cond. work index"() -> (w230:i32)
        n239 = local read "Local tree ref"() -> (w229:refnum<vi>)
        n240 = local write "Specifier(s)"(w248) -> ()
        n241 = Bundle By Name(cluster=w249, "Enabled"=w250, "Name"=w251, "Specifier(s)"=w248, "Response"=w252) -> (w246:T5)
        n242 = local read "Calibration parameters"() -> (w244:T13)
        n243 = local write "Subcondition"(w246) -> ()
        n244 = Replace Array Subset(array=w247, new element=w246, index=w230) -> (w245:T12)
        n245 = call "SW_Generate_Full_Condition(s)_text.vi"("Array index to show"=w230, "error in (no error)"=w243, "Array of conditions in"=w245, "Calibration parameters"=w244, "TreeControl ref in"=w229) -> ("error out"=w242:errorcluster)  [unwired: 5 in, 1 out]
        n246 = local write "Array of conditions out"(w245) -> ()
      }
      event "Save and exit": Value Change {
        n247 = event-data() -> ("OldVal"=w280:bool)  [unwired: 1 in, 5 out]
        n248 = local write "Save and exit"(w280) -> ()
        n249 = local read "Array of conditions out"() -> (w277:T12)
        n250 = local read "Array of conditions in"() -> (w278:T12)
        n251 = for {
          tunnel: w278 -> [w284] mode=indexing
          tunnel: w277 -> [w283] mode=indexing
          tunnel: [w282] -> w276 mode=indexing
          n252 = Not Equal?(x=w284, y=w283) -> (x != y?=w281:bool)
          n253 = case shown="True" w281 {
            tunnel: w283 -> [w285 w288]
            tunnel: [w285 w286] -> w282
            frame False {
            }
            frame True {
              n254 = Bundle By Name(cluster=w288, "Has been set"=TRUE) -> (w286:T5)
            }
          }
        }
        n255 = local write "Array of conditions out"(w276) -> ()
      }
      event "Reset Button": Value Change {
        n256 = event-data() -> ("OldVal"=w292:bool)  [unwired: 1 in, 5 out]
        n257 = local read "Array of conditions in"() -> (w289:T12)
        n258 = local write "Reset Button"(w292) -> ()
        n259 = local read "Subcondition #"() -> (w291:i32)
        n260 = Index Array(array=w289) -> ()  [unwired: 1 in, 1 out]
        n261 = local write "Array of conditions out"(w289) -> ()
        n262 = local read "Specifier(s)"() -> (w308:T11)
        n263 = Decrement(x=w291) -> (x-1=w293:i32)
        n264 = Index Array(array=w308, index=w293) -> (element=w307:T20)
        n265 = local read "Specifiers On/Off"() -> (w298:T2)
        n266 = Unbundle By Name(w307) -> ("Specifier enabled"=w294:bool, "Condition type"=w290:T6, "Comparison type"=w306:T7, "Value"=w305:dbl, "Validity criteria(s)"=w304:T4)
        n267 = Cluster To Array(cluster=w298) -> (array=w297:bool[])
        n268 = Replace Array Subset(array=w297, new element=w294, index=w293) -> (w296:bool[])
        n269 = Index Array(array=w304, index=0) -> (element=w302:T21)
        n270 = local write "SubCondition type"(w290) -> ()
        n271 = local write "Comparison type"(w306) -> ()
        n272 = local write "Compare against"(w305) -> ()
        n273 = Array To Cluster(array=w296) -> (cluster=w295:T22)
        n274 = Unbundle By Name(w302) -> ("V. check enabled"=w300:bool, "Criteria"=w301:T3, "Validity value"=w299:dbl)
        n275 = local write "Specifiers On/Off"(w295) -> ()
        n276 = local write "Validity Enabled"(w300) -> ()
        n277 = local write "SC. Validity Criteria"(w301) -> ()
        n278 = local write "Valid for, units"(w299) -> ()
      }
      event "Discard and exit": Value Change {
        n279 = event-data() -> ("OldVal"=w311:bool)  [unwired: 1 in, 5 out]
        n280 = local write "Discard and exit"(w311) -> ()
        n281 = local read "Array of conditions in"() -> (w309:T12)
        n282 = local write "Array of conditions out"(w309) -> ()
      }
    }
  }
  "error out" <- w16
